vi "Calculate Percent of Element.vi"(8 "error in (no error)":errorcluster caption="错误输入（无错误）", 11 "Gradient PieChart 输入":refnum<class "Gradient PieChart.lvclass"> caption="DNL_LabVIEW Object in") -> (0 "error out":errorcluster caption="错误输出", 1 "Angle":i16[](array[numeric]), 2 "Percent":dbl[](array[numeric]), 3 "Gradient PieChart 输出":refnum<class "Gradient PieChart.lvclass"> caption="DNL_LabVIEW Object out")   [LabVIEW 2012, in "Gradient PieChart.lvclass"]
uses:
  Gradient PieChart.lvclass
  Gradient PieChart.lvclass/Gradient PieChart.ctl
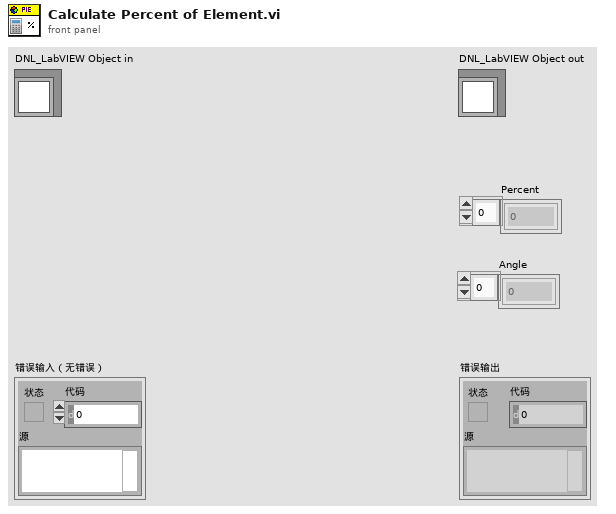
[diagram p1: front panel]
types:
  T1 = typedef "Gradient PieChart.lvclass/Info.ctl" = cluster{"Value":dbl, "Name":string, "NameTxtColor":u32, "Color Segement":u32[]}
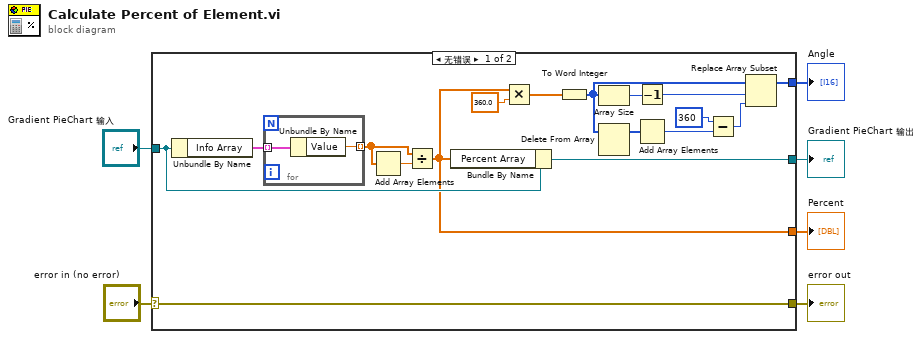
[diagram p0: block diagram]
diagram:
  n1 = case shown="无错误" "error in (no error)" {
    selector: "error in (no error)" -> [w23 w27]
    tunnel: [w23 w27] -> w5
    tunnel: [w18 w26] -> w3
    tunnel: "Gradient PieChart 输入" -> [w19 w26]
    tunnel: [w8 _] -> w2
    tunnel: [w7 _] -> w1
    frame No Error {
      n2 = Unbundle By Name(w19) -> ("Info Array"=w22:T1[])
      n3 = for {
        tunnel: w22 -> [w25] mode=indexing
        tunnel: [w24] -> w20 mode=indexing
        n4 = Unbundle By Name(w25) -> ("Value"=w24:dbl)
      }
      n5 = Add Array Elements(numeric array=w20) -> (sum=w21:dbl)
      n6 = Divide(x=w20, y=w21) -> (x/y=w8:dbl[])
      n7 = Bundle By Name(cluster=w19, "Percent Array"=w8) -> (w18:refnum<class "Gradient PieChart.lvclass">)
      n8 = Multiply(x=w8, y=360.0) -> (x*y=w10:dbl[])
      n9 = To Word Integer(number=w10) -> (16bit integer=w17:i16[])
      n10 = Array Size(array=w17) -> (size(s)=w14:i32)
      n11 = Delete From Array(array=w17) -> (array with subset deleted=w16:i16[])  [unwired: 2 in, 1 out]
      n12 = Decrement(x=w14) -> (x-1=w15:i32)
      n13 = Add Array Elements(numeric array=w16) -> (sum=w11:i16)
      n14 = Subtract(x=i16 360, y=w11) -> (x-y=w13:i16)
      n15 = Replace Array Subset(array=w17, new element=w13, index=w15) -> (w7:i16[])
    }
    frame Error {
    }
  }
  "error out" <- w5
  "Gradient PieChart 输出" <- w3
  "Percent" <- w2
  "Angle" <- w1
